vi "swabian_initialize.vi"(8 "error in (no error)":errorcluster, 11 "swabian_local_data_IN":T1={"events"={"update_status"=refnum, "update_chart"=refnum, "update_xy"=refnum, "send_channel_data"=refnum}, "stop_q"=refnum, "tagger_reference"=refnum, "connect_button"=refnum, "counter_reference"=refnum, "tagger_stream_reference"=refnum, "log_reference"=refnum, "current_log_offset"=0, "tt20_buffer_q"=refnum, "stream_to_file_button"=refnum, "num_records"=0, "connected?"=FALSE, "plots"=refnum, "histogram_bin_edges"=[], "histogrammer"=refnum, "plot_lifetimes"=refnum, "xy_graph"=refnum, "Reference\nChannel"=enum."ch0", "trigger_channels"=[], "filter_channels"=[], "active_channels"=[], "acq_mode"=0, "Reference\nChannel"=enum."ch0", "acq_time"=0, "sync_period_ps"=0, "raw_stream_path"=path "", "Leftovers"={"missing_sync_data"=[], "missing_events"=0}, "first_batch"=0, "first_sync_stamp"=0, "lifetime_settings"={"Plot Lifetimes"=FALSE, "start_time"=0.0, "stop_time"=0.0, "n_bins"=0}, "Histogram_bins"=[], "last_processed_data"=[], "histogram_data"=[]}) -> (0 "error out":errorcluster, 3 "swabian_local_data":T1={"events"={"update_status"=refnum, "update_chart"=refnum, "update_xy"=refnum, "send_channel_data"=refnum}, "stop_q"=refnum, "tagger_reference"=refnum, "connect_button"=refnum, "counter_reference"=refnum, "tagger_stream_reference"=refnum, "log_reference"=refnum, "current_log_offset"=0, "tt20_buffer_q"=refnum, "stream_to_file_button"=refnum, "num_records"=0, "connected?"=FALSE, "plots"=refnum, "histogram_bin_edges"=[], "histogrammer"=refnum, "plot_lifetimes"=refnum, "xy_graph"=refnum, "Reference\nChannel"=enum."ch0", "trigger_channels"=[], "filter_channels"=[], "active_channels"=[], "acq_mode"=0, "Reference\nChannel"=enum."ch0", "acq_time"=0, "sync_period_ps"=0, "raw_stream_path"=path "", "Leftovers"={"missing_sync_data"=[], "missing_events"=0}, "first_batch"=0, "first_sync_stamp"=0, "lifetime_settings"={"Plot Lifetimes"=FALSE, "start_time"=0.0, "stop_time"=0.0, "n_bins"=0}, "Histogram_bins"=[], "last_processed_data"=[], "histogram_data"=[]})   [LabVIEW 2018]
uses:
  swabian_local_data_tdef.ctl
  swabian_events_tdef.ctl
  update_chart_tdef.ctl
  channel_data_tdef.ctl
  C:/Users/bspoka/Documents/swabian_LV/lib/TTCSharp32.dll
  lib/TTCSharp32.dll
  swabian_buffer_tdef.ctl
  reference_checkbox_tdef.ctl
  lifetime_settings.ctl
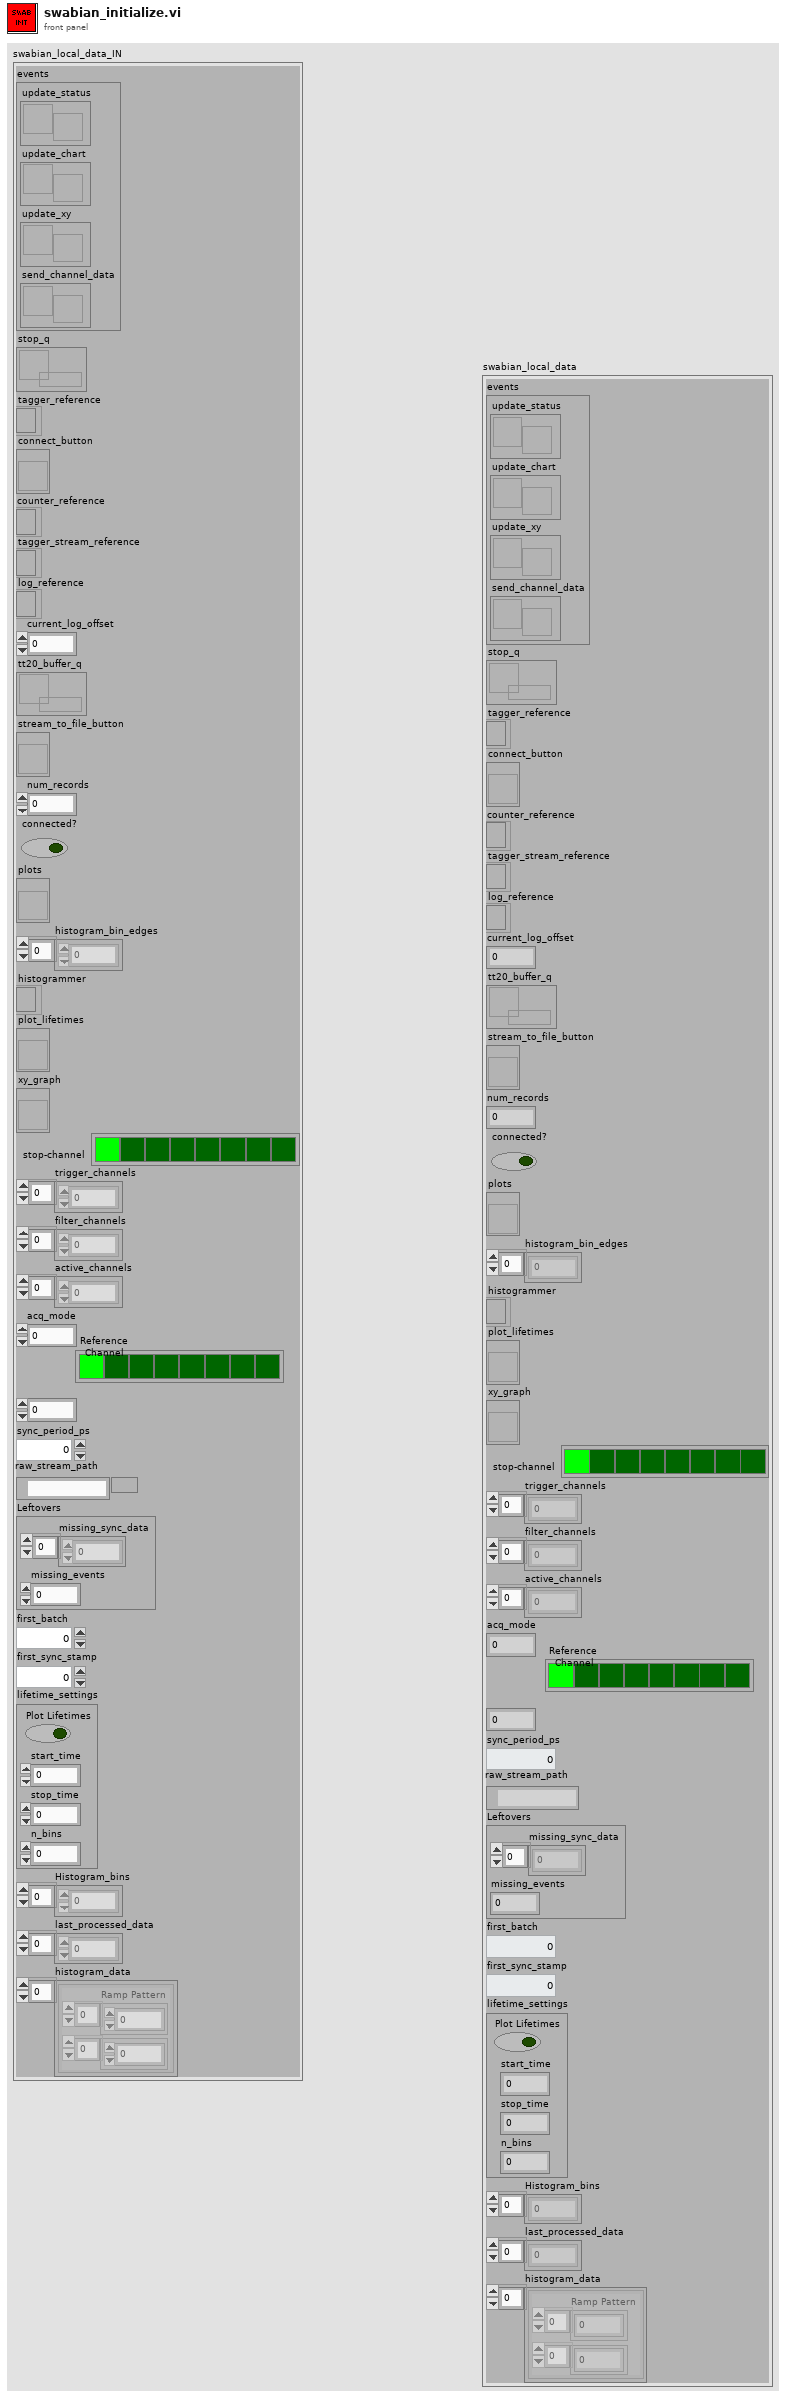
[diagram p1: front panel]
types:
  T1 = typedef "swabian_local_data_tdef.ctl" = cluster{"events":T2, "stop_q":refnum<queue>, "tagger_reference":refnum<k24>, "connect_button":refnum<vi>, "counter_reference":refnum<k24>, "tagger_stream_reference":refnum<k24>, "log_reference":refnum<file>, "current_log_offset":i64, "tt20_buffer_q":refnum<queue>, "stream_to_file_button":refnum<vi>, "num_records":u64, "connected?":bool, "plots":refnum<vi>, "histogram_bin_edges":i64[], "histogrammer":refnum<k24>, "plot_lifetimes":refnum<vi>, "xy_graph":refnum<vi>, "Reference\nChannel":T3, "trigger_channels":i32[], "filter_channels":i32[], "active_channels":i32[], "acq_mode":i32, "Reference\nChannel":T3, "acq_time":i64, "sync_period_ps":i64, "raw_stream_path":path, "Leftovers":cluster{"missing_sync_data":i64[], "missing_events":i32}, "first_batch":i32, "first_sync_stamp":i64, "lifetime_settings":T4, "Histogram_bins":dbl[], "last_processed_data":i64[], "histogram_data":cluster{"Ramp Pattern":dbl[], dbl[]}[]}
  T2 = typedef "swabian_events_tdef.ctl" = cluster{"update_status":refnum<user-event>, "update_chart":refnum<user-event>, "update_xy":refnum<user-event>, "send_channel_data":refnum<user-event>}
  T3 = typedef "reference_checkbox_tdef.ctl" = enum32{"No Selection", "ch0", "ch1", "ch2", "ch3", "ch4", "ch5", "ch6", "ch7"}
  T4 = typedef "lifetime_settings.ctl" = cluster{"Plot Lifetimes":bool, "start_time":dbl, "stop_time":dbl, "n_bins":i32}
  T5 = enum8{"Enabled", "Disabled", "Disabled and Grayed Out"}
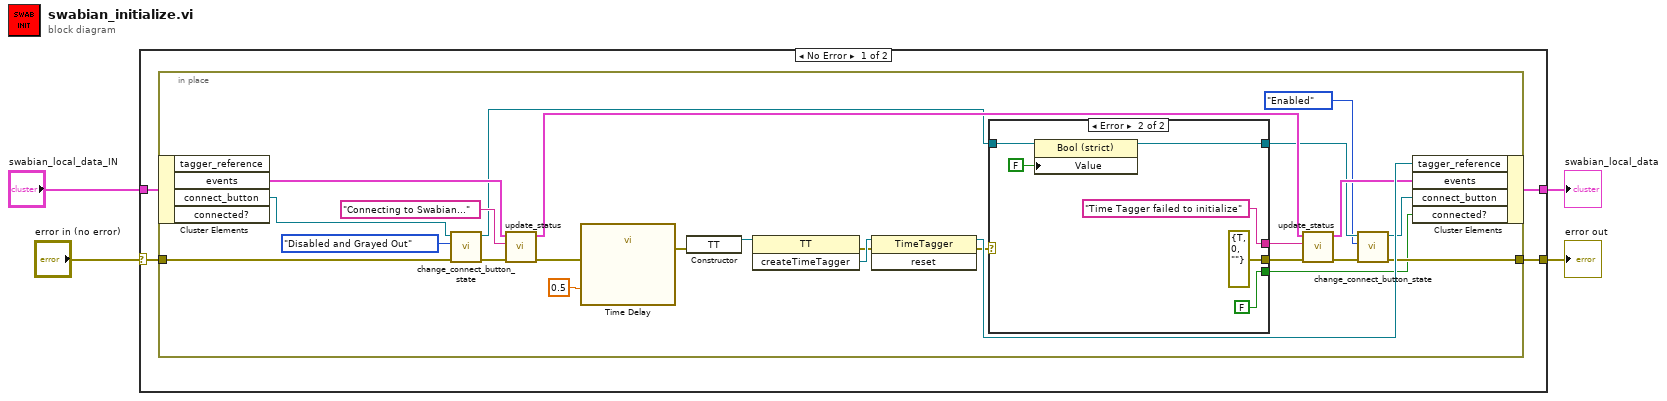
[diagram p0: block diagram]
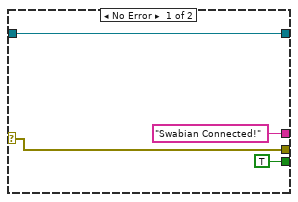
[diagram p2: hidden frame]
diagram:
  n1 = case shown="No Error" "error in (no error)" {
    selector: "error in (no error)" -> [w7 w45]
    tunnel: "swabian_local_data_IN" -> [w8 w44]
    tunnel: [w6 w45] -> w2
    tunnel: [w5 w44] -> w1
    frame No Error {
      n2 = in-place {
        in-place-border: w7 -> [w19]
        in-place-border: [w22] -> w6
        n3 = in-place-cluster #1(w8) -> ("events"=w29:T2, "connect_button"=w16:refnum<vi>)  [unwired: 2 out]
        n4 = call "change_connect_button_state.vi"("error in (no error)"=w19, "button_status"=T5."Disabled and Grayed Out" ("Disabled"), "Boolean in"=w16) -> ("error out"=w18:errorcluster, "Boolean out"=w15:refnum<vi>)  [unwired: 7 in]
        n5 = call "update_status.vi"("error in (no error)"=w18, "status"="Connecting to Swabian...", "events"=w29) -> ("error out"=w25:errorcluster, "events_out"=w28:T2)  [unwired: 7 in]
        n6 = call "Time Delay"("error in (no error)"=w25, "Delay Time (s)"=0.5) -> ("error out"=w12:errorcluster)  [unwired: 9 in]
        n7 = constructor class="TT"(error in=w12) -> (reference out=w11:refnum<k24>)  [unwired: 2 in, 2 out]
        n8 = invoke class="TT" method="createTimeTagger"(reference=w11) -> (error out=w9:errorcluster, "createTimeTagger"=w10:refnum<k24>)  [unwired: 2 in, 1 out]
        n9 = invoke class="TimeTagger" method="reset"(reference=w10, error in=w9) -> (reference out=w33:refnum<k24>, error out=w13:errorcluster)  [unwired: 1 in, 1 out]
        n10 = case shown="Error" w13 {
          selector: w13 -> [w36 _]
          tunnel: [w36 errorcluster {"status"=TRUE, "code"=0, "source"=""} ("error IO")] -> w32
          tunnel: ["Swabian Connected!" ("source") "Time Tagger failed to initialize" ("source")] -> w30
          tunnel: w15 -> [w35 w40]
          tunnel: [w35 w39] -> w21
          tunnel: [TRUE FALSE] -> w14
          frame No Error {
          }
          frame Error {
            n11 = property class="Bool (strict)"(reference=w40, "Value"=FALSE) -> (reference out=w39:refnum<vi>)  [unwired: 1 in, 1 out]
          }
        }
        n12 = call "update_status.vi"("error in (no error)"=w32, "status"=w30, "events"=w28) -> ("error out"=w23:errorcluster, "events_out"=w31:T2)  [unwired: 7 in]
        n13 = call "change_connect_button_state.vi"("error in (no error)"=w23, "button_status"=T5."Enabled", "Boolean in"=w21) -> ("error out"=w22:errorcluster, "Boolean out"=w24:refnum<vi>)  [unwired: 7 in]
        n14 = in-place-cluster #1("tagger_reference"=w33, "events"=w31, "connect_button"=w24, "connected?"=w14) -> (w5:T1)
      }
    }
    frame Error {
    }
  }
  "error out" <- w2
  "swabian_local_data" <- w1
